vi "Rising_Edge.vi"(11 "input":bool) -> (3 "rising_edge":bool)   [LabVIEW 2021]
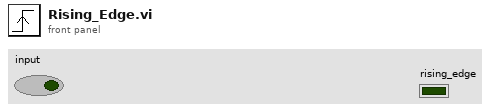
[diagram p1: front panel]
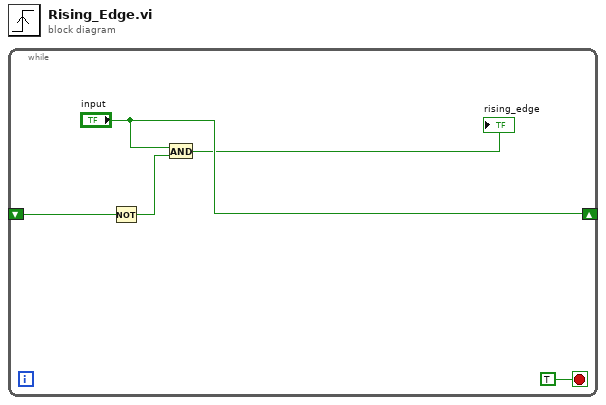
[diagram p0: block diagram]
diagram:
  n1 = while {
    shift-right: ["input"] -> _
    shift-left: _ -> [w1]
    stop <- TRUE stop-if-true
    n2 = Not(x=w1) -> (.not. x?=w3:bool)
    n3 = And(x="input", y=w3) -> (x .and. y?=→"rising_edge":bool)
  }
